vi "mxwScript_API_XMLTemplateName_AddTargetRef.vi"(4 "relativeToExistData":T1, 6 "terminalData":T2={"name"="", "termIsTag"=FALSE, "referencePosition"=enum."Middle"}, 7 "targetRefType":T6, 8 "error in (no error)":errorcluster, 9 "absoluteData":T5, 10 "templateData":T3={"tag"="", "index"=-1, "targetRefTemplateType"=enum."OutputAverage", "referencePosition"=enum."Right", "terminalData"={"name"="", "termIsTag"=FALSE, "referencePosition"=enum."Middle"}}, 11 "absolutePath":string) -> (0 "error out":errorcluster, 3 "encoded absolutePath":string)   [LabVIEW 2020]
doc: "Add information to override the default method for locating the reference point on the block diagram during template drop."
uses:
  codeGenAPISupport.llb/cgAPI_mxwScript_DrpTmplt_TargetRefType.ctl
  codeGenAPISupport.llb/cgAPI_mxwScript_DrpTmplt_AbsoluteData.ctl
  codeGenAPISupport.llb/cgAPI_mxwScript_DrpTmplt_TargetRefTemplateData.ctl
  codeGenAPISupport.llb/cgAPI_mxwScript_DrpTmplt_TargetRefTemplateType.ctl
  codeGenAPISupport.llb/cgAPI_mxwScript_DrpTmplt_ReferencePosition.ctl
  codeGenAPISupport.llb/cgAPI_mxwScript_DrpTmplt_TerminalData.ctl
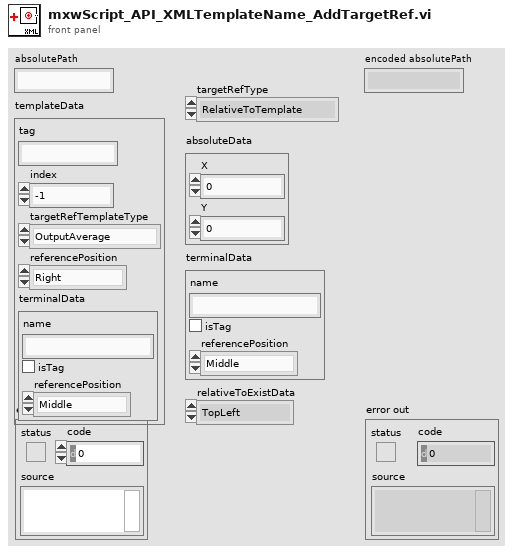
[diagram p1: front panel]
types:
  T1 = typedef "cgAPI_mxwScript_DrpTmplt_ReferencePosition.ctl" = enum16{"TopLeft", "Top", "TopRight", "Left", "Middle", "Right", "BottomLeft", "Bottom", "BottomRight"}
  T2 = typedef "cgAPI_mxwScript_DrpTmplt_TerminalData.ctl" = cluster{"name":string, "termIsTag":bool, "referencePosition":T1}
  T3 = typedef "cgAPI_mxwScript_DrpTmplt_TargetRefTemplateData.ctl" = cluster{"tag":string, "index":i32, "targetRefTemplateType":T4, "referencePosition":T1, "terminalData":T2}
  T4 = typedef "cgAPI_mxwScript_DrpTmplt_TargetRefTemplateType.ctl" = enum16{"OutputAverage", "Absolute", "Terminal"}
  T5 = typedef "cgAPI_mxwScript_DrpTmplt_AbsoluteData.ctl" = cluster{"X":i32, "Y":i32}
  T6 = typedef "cgAPI_mxwScript_DrpTmplt_TargetRefType.ctl" = enum16{"RelativeToTemplate", "RelativeToTerminal", "AbsoluteOnRoot", "AbsoluteOnTarget", "RelativeToExistOnRoot"}
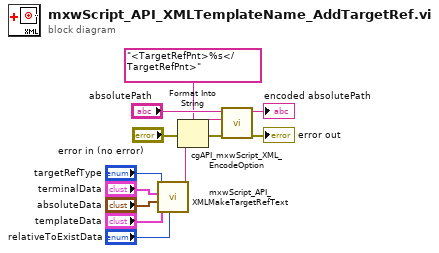
[diagram p0: block diagram]
diagram:
  n1 = call "mxwScript_API_XMLMakeTargetRefText.vi"("relativeToExistData"="relativeToExistData", "templateData"="templateData", "absoluteData"="absoluteData", "terminalData"="terminalData", "targetRefType"="targetRefType") -> ("targetRefText"=w6:string)  [unwired: 6 out]
  n2 = Format Into String(format string="<TargetRefPnt>%s</TargetRefPnt>" ("control name"), error in="error in (no error)", w6) -> (resulting string=w8:string, error out=w10:errorcluster)  [unwired: 1 in]
  n3 = call "cgAPI_mxwScript_XML_EncodeOption.vi"("error in (no error)"=w10, "otherXML"=w8, "normalTextString"="absolutePath") -> ("error out"=→"error out":errorcluster, "encodedString"=→"encoded absolutePath":string)  [unwired: 7 out]
